vi "NormStr2HexStr.vi"(1 "string":string) -> (0 "hex string":string)   [LabVIEW 2013]
doc: "Converts normal string to hex string\n\n\nby: ian f koo\nemail: labview@ianfung.net\ndate: 08/2003"
panel:
  out "substring":string
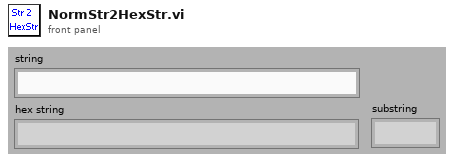
[diagram p1: front panel]
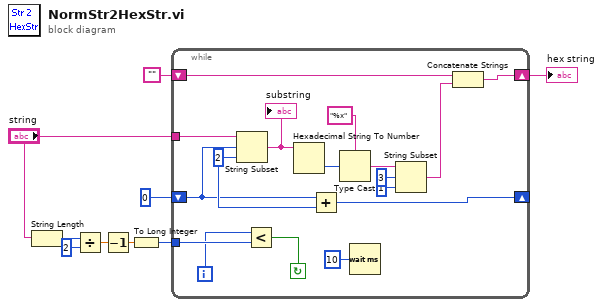
[diagram p0: block diagram]
diagram:
  n1 = String Length(string="string") -> (length=w8:i32)
  n2 = Divide(x=w8, y=2) -> (x/y=w6:dbl)
  n3 = Decrement(x=w6) -> (x-1=w4:dbl)
  n4 = To Long Integer(number=w4) -> (32bit integer=w3:i32)
  n5 = while {
    tunnel: "string" -> [w26]
    tunnel: w3 -> [w21]
    shift-right: [w17] -> _
    shift-left: 0 ("length (rest)") -> [w16]
    shift-right: [w13] -> w1
    shift-left: "" -> [w14]
    i -> [w18]
    stop <- w20 continue-if-true
    w19 = 2 ("length (rest)")
    n6 = String Subset(string=w26, offset (0)=w16, length (rest)=w19) -> (substring=w24:string)
    "substring" <- w24
    n7 = Less?(x=w18, y=w21) -> (x < y?=w20:bool)
    n8 = Hexadecimal String To Number(string=w24) -> (number=w25:u32)  [unwired: 2 in, 1 out]
    n9 = Add(x=w16, y=w19) -> (x+y=w17:i32)
    n10 = Type Cast(type="%x", x=w25) -> (*(type *) &x=w23:string)
    n11 = Wait (ms)(milliseconds to wait=u32 10) -> ()  [unwired: 1 out]
    n12 = String Subset(string=w23, offset (0)=3, length (rest)=1 ("length (rest)")) -> (substring=w22:string)
    n13 = Concatenate Strings(w14, w22) -> (w13:string)
  }
  "hex string" <- w1
